vi "Create Measurement Services.vi"(8 "error in":errorcluster, 10 "measurement service versions":T1[](array[typedef]), 11 "gRPC ID in":T2) -> (0 "error out":errorcluster, 2 "measurement service array out":refnum<class "IMeasurement Service.lvclass">[](array[class]), 3 "gRPC ID out":T2)   [LabVIEW 2021, in "NI Measurement Plug-In SDK.lvlib"]
uses:
  NI Measurement Plug-In SDK.lvlib
  IMeasurement Service/IMeasurement Service.lvclass
  <vilib>/gRPC/LabVIEW gRPC Library/Shared/grpcId.ctl
  TypeDefs/Measurement Service Version.ctl
  Measurement Service V2/Measurement Service V2.lvclass
  Measurement Service V1/Measurement Service V1.lvclass
  <vilib>/gRPC/LabVIEW gRPC Library/grpc-lvsupport-release.lvlib
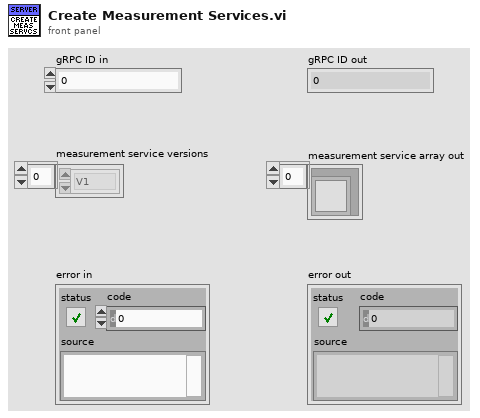
[diagram p1: front panel]
types:
  T1 = typedef "NI Measurement Plug-In SDK.lvlib/Measurement Service Version.ctl" = enum16{"V1", "V2"}
  T2 = typedef "grpc-lvsupport-release.lvlib/grpcId.ctl" = u64
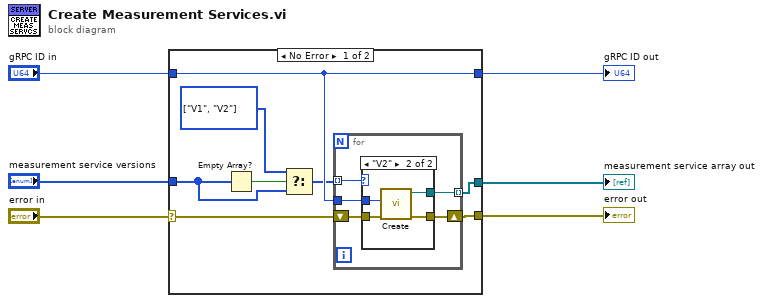
[diagram p0: block diagram]
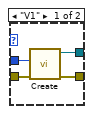
[diagram p2: hidden frame]
diagram:
  n1 = case shown="No Error" "error in" {
    selector: "error in" -> [w13 w29]
    tunnel: [w14 w29] -> w5
    tunnel: [w12 _] -> w4
    tunnel: "gRPC ID in" -> [w11 w28]
    tunnel: [w11 w28] -> w2
    tunnel: "measurement service versions" -> [w8 _]
    frame No Error {
      w7 = T1[] [enum."V1", enum."V2"] items=["V1", "V2"]
      n2 = Empty Array?(array=w8) -> (empty?=w10:bool)
      n3 = Select(t=w7, s=w10, f=w8) -> (s? t:f=w9:T1[])
      n4 = for {
        tunnel: [w15] -> w12 mode=indexing
        tunnel: w11 -> [w18]
        shift-right: [w16] -> w14
        shift-left: w13 -> [w19]
        tunnel: w9 -> [w17] mode=indexing
        n5 = case shown="\"V2\"" w17 {
          tunnel: w19 -> [w22 w26]
          tunnel: w18 -> [w23 w27]
          tunnel: [w21 w25] -> w16
          tunnel: [w20 w24] -> w15
          frame "V1" {
            n6 = call "Create.vi"("error in"=w22, "gRPC ID in"=w23) -> ("error out"=w21:errorcluster, "measurement service out"=w20:refnum<class "IMeasurement Service.lvclass">)  [unwired: 7 in, 1 out]
          }
          frame "V2" {
            n7 = call "Create.vi"("error in"=w26, "gRPC ID in"=w27) -> ("error out"=w25:errorcluster, "measurement service out"=w24:refnum<class "IMeasurement Service.lvclass">)  [unwired: 7 in, 1 out]
          }
        }
      }
    }
    frame Error {
    }
  }
  "error out" <- w5
  "measurement service array out" <- w4
  "gRPC ID out" <- w2
